vi "读取数据库.vi"(5 "精度(6)":i16=2, 7 "condition":string, 8 "error in (no error)":errorcluster caption="错误输入（无错误）", 9 "database":string="database1.mdb", 10 "显示项":string[](array[string]), 11 "组合框":string(combo)) -> (0 "error out":errorcluster caption="错误输出", 1 "columns":string[](array[string]), 2 "data":variant[][](array[variant]), 3 "表格":string[][](table))   [LabVIEW 2016]
uses:
  <vilib>/Utility/sysdir.llb/System Directory Type.ctl
  <vilib>/addons/database/Connection.llb/DB Tools Open Connec (String).vi
  <vilib>/addons/database/_DB Variant To Data/Database Variant To Data.xnode
  <vilib>/addons/database/NI_Database_API.lvlib
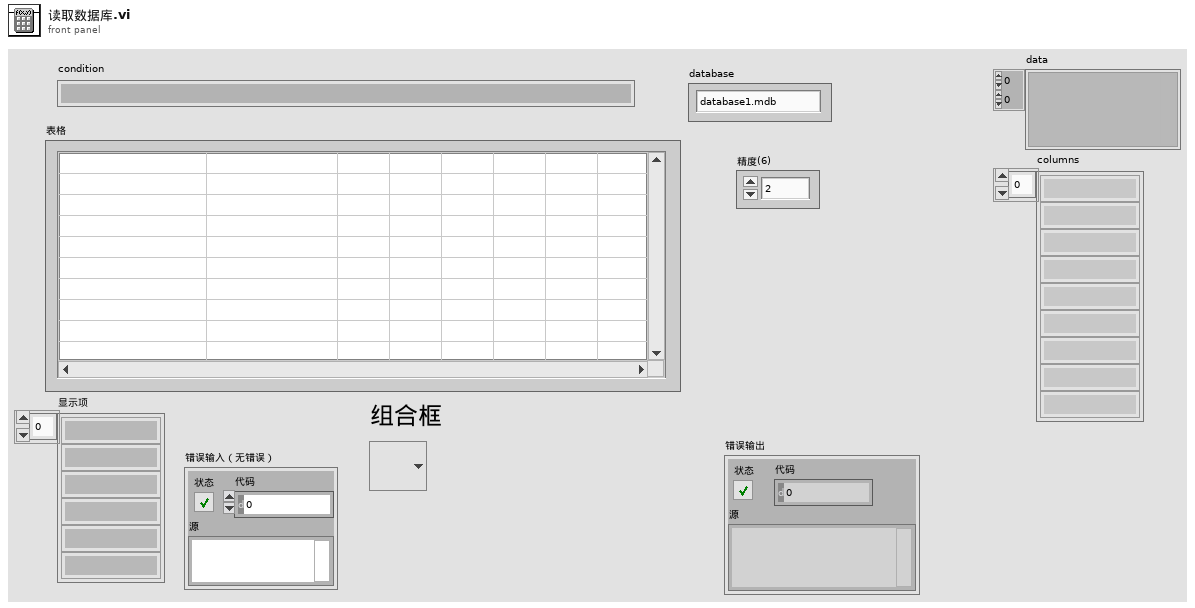
[diagram p1: front panel]
types:
  T1 = typedef "System Directory Type.ctl" = i32
  T2 = typedef "NI_Database_API.lvlib/Conn ObjectReference.ctl" = refnum<k1>
  T3 = typedef "NI_Database_API.lvlib/DB Tools DataTypes.ctl" = enum16{"String", "Long (I32)", "Single (SGL)", "Double (DBL)", "Date/Time", "Binary"}
  T4 = cluster{"name":string, "database data type":T3, "defined size":i32}[]
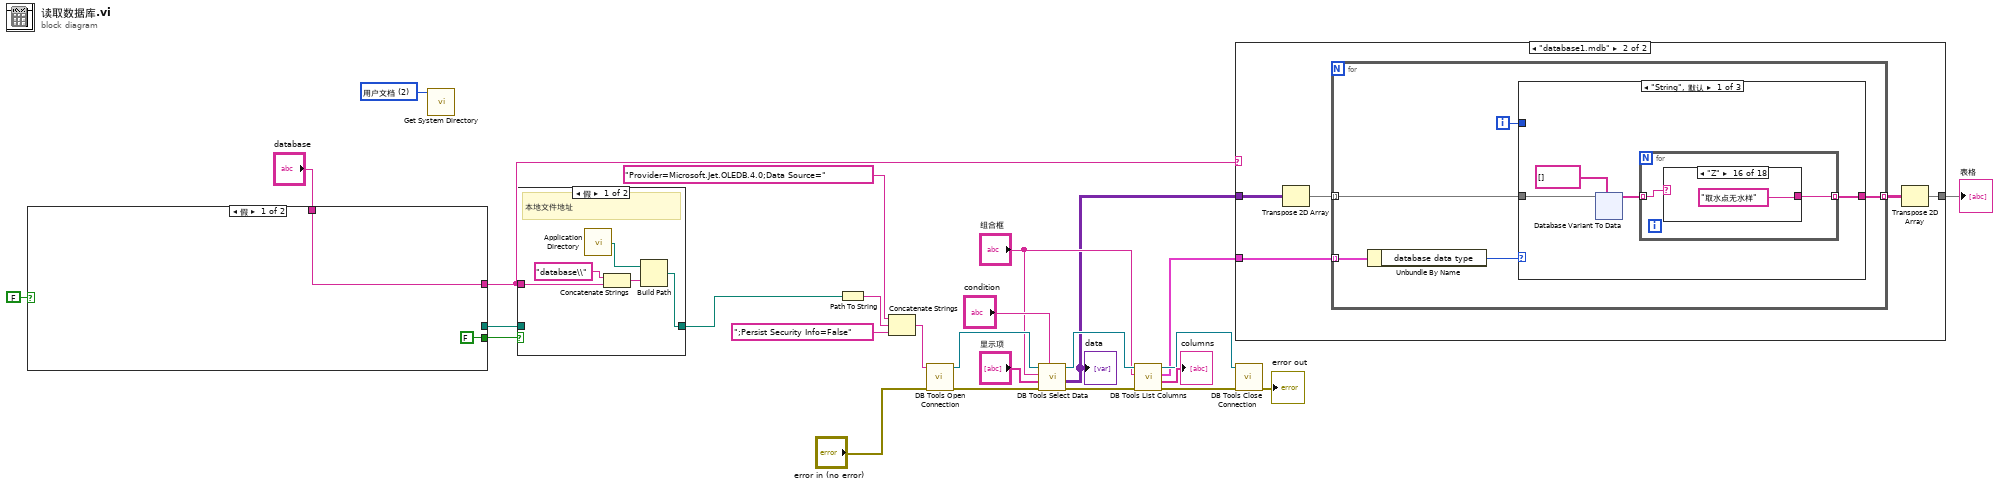
[diagram p0: block diagram]
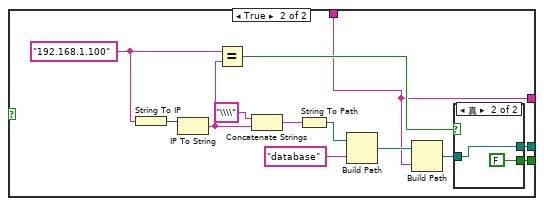
[diagram p2: hidden frame]
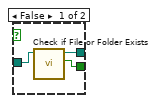
[diagram p3: hidden frame]
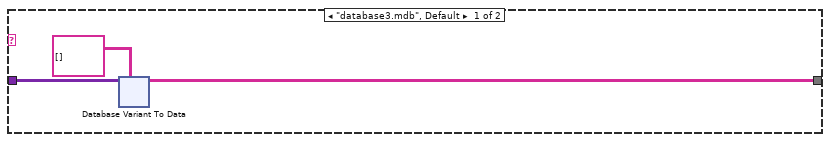
[diagram p5: hidden frame]
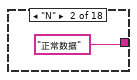
[diagram p7: hidden frame]
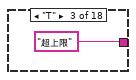
[diagram p8: hidden frame]
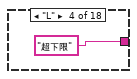
[diagram p9: hidden frame]
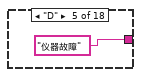
[diagram p10: hidden frame]
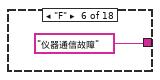
[diagram p11: hidden frame]
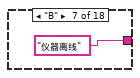
[diagram p12: hidden frame]
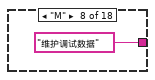
[diagram p13: hidden frame]
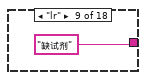
[diagram p14: hidden frame]
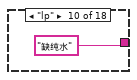
[diagram p15: hidden frame]
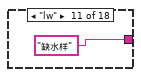
[diagram p16: hidden frame]
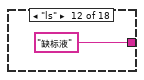
[diagram p17: hidden frame]
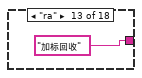
[diagram p18: hidden frame]
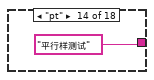
[diagram p19: hidden frame]
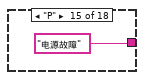
[diagram p20: hidden frame]
diagram:
  w1 = T1 2 items=["用户目录"=0, "用户桌面"=1, "用户文档"=2, "用户应用程序数据"=3, "用户设置"=4, "用户临时目录"=5, "公共文档"=6, "公共应用程序数据"=7, "公共设置"=8, "公共缓存"=13, "系统核心库"=9, "系统安装库"=10, "应用程序文件"=11, "启动盘根目录"=12] ("system directory type")
  n1 = case shown="假" FALSE {
    tunnel: [_ w32] -> w7
    tunnel: [FALSE ("file or folder exists?") w31] -> w6
    tunnel: [w27 w29] -> w4
    tunnel: "database" -> [w27 w29]
    frame False {
    }
    frame True {
      w30 = "192.168.1.100" ("名称")
      n2 = String To IP(1:w30) -> (0:w41:u32)
      n3 = IP To String(2:w41) -> (0:w35:string)  [unwired: 1 in]
      n4 = Equal?(x=w30, y=w35) -> (x = y?=w34:bool)
      n5 = Concatenate Strings("\\\\" ("字符串"), w35) -> (w38:string)
      n6 = String To Path(string=w38) -> (path=w40:path)
      n7 = Build Path(base path=w40, name or relative path="database" ("名称或相对路径")) -> (appended path=w36:path)
      n8 = Build Path(base path=w36, name or relative path=w29) -> (appended path=w33:path)
      n9 = case shown="真" w34 {
        tunnel: w33 -> [w44 w45]
        tunnel: [w43 w45] -> w32
        tunnel: [w42 FALSE] -> w31
        frame False {
          n10 = call <vilib>:"Check if File or Folder Exists.vi"("path"=w44) -> ("file or folder exists?"=w42:bool, "dup path"=w43:path)  [unwired: 8 in, 1 out]
        }
        frame True {
        }
      }
    }
  }
  n11 = call <vilib>:"Get System Directory.vi"("system directory type"=w1) -> ()  [unwired: 10 in, 1 out]
  n12 = case shown="假" w6 {
    tunnel: w4 -> [w49 _]
    tunnel: w7 -> [_ w52]
    tunnel: [w48 w52] -> w5
    frame False {
      # "本地文件地址"
      n13 = call <vilib>:"Application Directory.vi"() -> ("Application Directory"=w47:path)
      n14 = Concatenate Strings("database\\" ("名称或相对路径"), w49) -> (w50:string)
      n15 = Build Path(base path=w47, name or relative path=w50) -> (appended path=w48:path)
    }
    frame True {
      # "网络共享地址"
    }
  }
  n16 = Path To String(path=w5) -> (string=w13:string)
  n17 = Concatenate Strings("Provider=Microsoft.Jet.OLEDB.4.0;Data Source=", w13, ";Persist Security Info=False") -> (w12:string)
  n18 = call-poly <vilib>:"DB Tools Open Connection.vi"("error in (no error)"="error in (no error)", "connection information"=w12) -> ("error out"=w25:errorcluster, "connection reference"=w26:T2)  [unwired: 6 in]
  n19 = call <vilib>:"DB Tools Select Data.vi"("condition"="condition", "error in (no error)"=w25, "columns"="显示项", "table"="组合框", "connection reference"=w26) -> ("error out"=w24:errorcluster, "data"=w10:variant[][], "connection reference out"=w21:T2)  [unwired: 1 in]
  "data" <- w10
  n20 = call <vilib>:"DB Tools List Columns.vi"("error in (no error)"=w24, "table"="组合框", "connection reference"=w21) -> ("error out"=w16:errorcluster, "columns"=→"columns":string[], "column information"=w9:T4, "connection reference out"=w17:T2)  [unwired: 1 in]
  n21 = case shown="\"database1.mdb\"" w4 {
    tunnel: w10 -> [w54 w104]
    tunnel: w9 -> [_ w102]
    tunnel: [w53 w100] -> w8
    frame "database3.mdb", Default {
      n22 = xnode "Database Variant To Data"("database variant"=w54, "type"=string[][] []) -> ("data"=w53:string[][])  [unwired: 1 in, 1 out]
    }
    frame "database1.mdb" {
      n23 = Transpose 2D Array(2D array=w104) -> (transposed array=w103:variant[][])
      n24 = for {
        tunnel: w103 -> [w107] mode=indexing
        tunnel: w102 -> [w109] mode=indexing
        tunnel: [w106] -> w101 mode=indexing
        i -> [w105]
        n25 = Unbundle By Name(w109) -> ("database data type"=w108:T3)
        n26 = case shown="\"String\", 默认" w108 {
          tunnel: w107 -> [w112 w174 w265]
          tunnel: [w110 w173 w263] -> w106
          tunnel: w105 -> [_ w172 _]
          frame "String", Default {
            n27 = xnode "Database Variant To Data"("database variant"=w112, "type"=string[] []) -> ("data"=w111:string[])  [unwired: 1 in, 1 out]
            n28 = for {
              tunnel: w111 -> [w115] mode=indexing
              tunnel: [w114] -> w110 mode=indexing
              n29 = case shown="\"Z\"" w115 {
                selector: w115 -> [w116 _ _ _ _ _ _ _ _ _ _ _ _ _ _ _ _ _]
                tunnel: [w116 "正常数据" "超上限" "超下限" "仪器故障" "仪器通信故障" "仪器离线" "维护调试数据" "缺试剂" "缺纯水" "缺水样" "缺标液" "加标回收" "平行样测试" "电源故障" "取水点无水样" "手工输入数据" "手动测试数据"] -> w114
                frame Default {
                }
                frame "N" {
                }
                frame "T" {
                }
                frame "L" {
                }
                frame "D" {
                }
                frame "F" {
                }
                frame "B" {
                }
                frame "M" {
                }
                frame "lr" {
                }
                frame "lp" {
                }
                frame "lw" {
                }
                frame "ls" {
                }
                frame "ra" {
                }
                frame "pt" {
                }
                frame "P" {
                }
                frame "Z" {
                }
                frame "S" {
                }
                frame "hd" {
                }
              }
            }
          }
          frame "Single (SGL)", "Double (DBL)" {
            n30 = case shown="默认" w172 {
              tunnel: w174 -> [w179 w220]
              tunnel: [w175 w218] -> w173
              frame 3 {
                n31 = xnode "Database Variant To Data"("database variant"=w179, "type"=dbl[] []) -> ("data"=w177:dbl[])  [unwired: 1 in, 1 out]
                n32 = Number To Fractional String(number=w177, precision (6)="精度(6)") -> (F-format string=w175:string[])  [unwired: 2 in]
              }
              frame Default {
                n33 = xnode "Database Variant To Data"("database variant"=w220, "type"=dbl[] []) -> ("data"=w219:dbl[])  [unwired: 1 in, 1 out]
                n34 = for {
                  tunnel: w219 -> [w224] mode=indexing
                  tunnel: [w222] -> w218 mode=indexing
                  n35 = Format Into String(format string="%#.4f" ("格式字符串"), w224) -> (resulting string=w222:string)  [unwired: 2 in, 1 out]
                }
              }
            }
          }
          frame "Date/Time" {
            n36 = xnode "Database Variant To Data"("database variant"=w265, "type"=timestamp[] []) -> ("data"=w264:timestamp[])  [unwired: 1 in, 1 out]
            n37 = for {
              tunnel: w264 -> [w268] mode=indexing
              tunnel: [w267] -> w263 mode=indexing
              n38 = Format Date/Time String(time format string (%c)="%y/%m/%d %H:%M:%S" ("时间格式字符串(%c)"), seconds (now)=w268) -> (date/time string=w267:string)  [unwired: 1 in]
            }
          }
        }
      }
      n39 = Transpose 2D Array(2D array=w101) -> (transposed array=w100:string[][])
    }
  }
  "表格" <- w8
  n40 = call <vilib>:"DB Tools Close Connection.vi"("error in (no error)"=w16, "connection reference"=w17) -> ("error out"=→"error out":errorcluster)  [unwired: 5 in]
